vi "JsonFile Save.vi"(8 "error in (no error)":errorcluster, 10 "JSON String":string, 11 "Path":path) -> (0 "error out":errorcluster)   [LabVIEW 2019, in "lv-apt-json-file.lvlib"]
uses:
  lv-apt-json-file.lvlib
  <vilib>/addons/_JKI.lib/Serialization/JSON/Library/Unflatten From JSON String.vi
  <vilib>/Utility/error.llb/Error Cluster From Error Code.vi
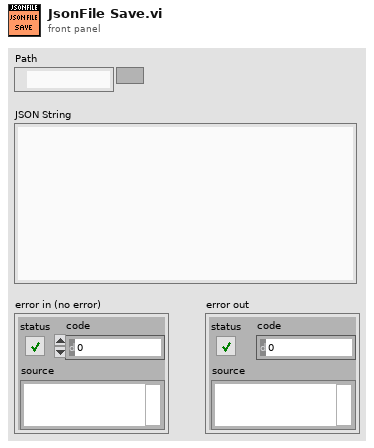
[diagram p1: front panel]
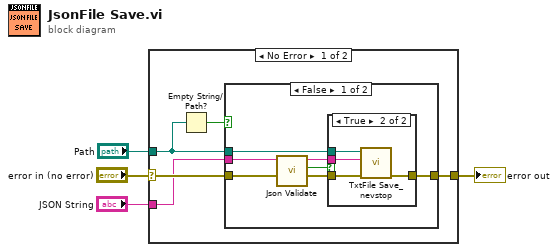
[diagram p0: block diagram]
diagram:
  n1 = case shown="No Error" "error in (no error)" {
    selector: "error in (no error)" -> [w7 w23]
    tunnel: [w9 w23] -> w4
    tunnel: "Path" -> [w6 _]
    tunnel: "JSON String" -> [w5 _]
    frame No Error {
      n2 = Empty String/Path?(string/path=w6) -> (empty?=w8:bool)
      n3 = case shown="False" w8 {
        tunnel: w7 -> [w12 w22]
        tunnel: [w16 w22] -> w9
        tunnel: w5 -> [w14 _]
        tunnel: w6 -> [w15 _]
        frame False {
          n4 = call "Json Validate.vi"("error in (no error)"=w12, "String"=w14) -> ("error out"=w11:errorcluster, "Valid Json?"=w10:bool, "String (dup)"=w13:string)  [unwired: 7 in]
          n5 = case shown="True" w10 {
            tunnel: [w17 w21] -> w16
            tunnel: w15 -> [_ w20]
            tunnel: w13 -> [_ w19]
            tunnel: w11 -> [w17 w18]
            frame False {
            }
            frame True {
              n6 = call <userlib>:"TxtFile Save_nevstop.vi"("error in (no error)"=w18, "text"=w19, "Path"=w20) -> ("error out"=w21:errorcluster)  [unwired: 8 in]
            }
          }
        }
        frame True {
        }
      }
    }
    frame Error {
    }
  }
  "error out" <- w4
